vi "GetProviderName.vi"(0 "ClassWriterGOOP300 in":refnum<class "ClassWriterGOOP400.lvclass">, 5 "error in (no error)":errorcluster) -> (14 "ClassWriterGOOP300 out":refnum<class "ClassWriterGOOP400.lvclass">, 15 "ProviderName":string, 17 "TranslatedProviderName":string, 18 "ShortName(Could be used in for INI Sections)":string, 19 "error out":errorcluster)   [LabVIEW 2020, in "ClassWriterGOOP400.lvclass"]
uses:
  <resource>/Framework/Providers/Open_GDS/ClassProviders/Provider_EndevoGOOP400/ClassWriterGOOP400_class/ClassWriterGOOP400.lvclass
  <resource>/Framework/Providers/Open_GDS/ClassProviders/Provider_EndevoGOOP400/EndevoG4ProviderName.ctl
  <resource>/Framework/Providers/Open_GDS/ClassProviders/Provider_EndevoGOOP400/ClassWriterGOOP400_class/ClassWriterGOOP400.lvclass/ClassWriterGOOP400.ctl
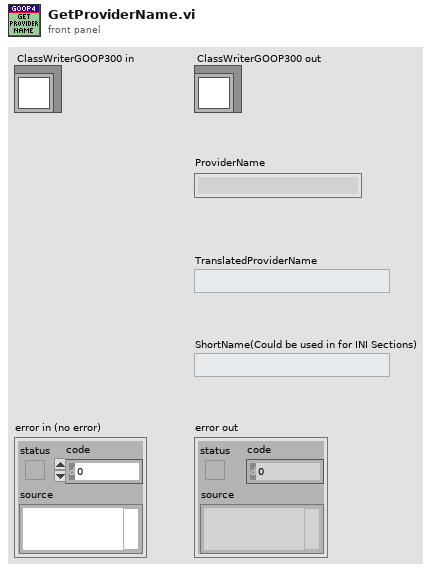
[diagram p1: front panel]
types:
  T1 = typedef "EndevoG4ProviderName.ctl" = enum16{"EndevoGOOP400"}
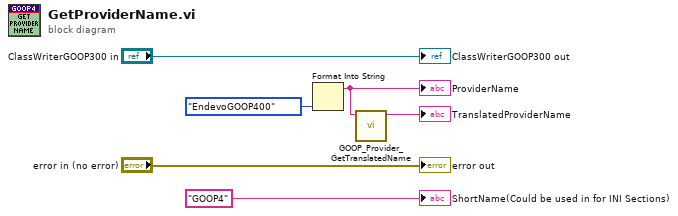
[diagram p0: block diagram]
diagram:
  n1 = Format Into String(EndevoG4ProviderName."EndevoGOOP400" ("ProviderName")) -> (resulting string=w3:string)  [unwired: 3 in, 1 out]
  "ProviderName" <- w3
  n2 = call <resource>:"GOOP_Provider_GetTranslatedName.vi"("ProviderName"=w3) -> ("TranslatedName"=→"TranslatedProviderName":string)  [unwired: 10 in]
  "ClassWriterGOOP300 out" <- "ClassWriterGOOP300 in"
  "error out" <- "error in (no error)"
  "ShortName(Could be used in for INI Sections)" <- "GOOP4" ("ClassType")
